vi "Add.vi"(8 "error in (no error)":errorcluster, 9 "Project":refnum<vi>, 10 "IB_Destination.lvclass":refnum<class "IB_Destination.lvclass">, 11 "IB_Tree_Item_Proj in":refnum<class "IB_Tree_Item_Proj.lvclass">) -> (0 "error out":errorcluster, 1 "updated?":bool, 2 "IB_Source.lvclass":refnum<class "IB_Source.lvclass">, 3 "IB_Tree_Item_Proj out":refnum<class "IB_Tree_Item_Proj.lvclass">)   [LabVIEW 2020, in "IB_Tree_Item_Proj.lvclass"]
uses:
  <vilib>/AppBuilder/IB_Classes/Tree_Item_Proj/IB_Tree_Item_Proj.lvclass
  <vilib>/AppBuilder/IB_Classes/Tree_Item_Proj/IB_Tree_Item_Proj.lvclass/IB_Tree_Item_Proj.ctl
  <vilib>/AppBuilder/IB_Classes/Source/IB_Source.lvclass
  <vilib>/AppBuilder/IB_Classes/Destination/IB_Destination.lvclass
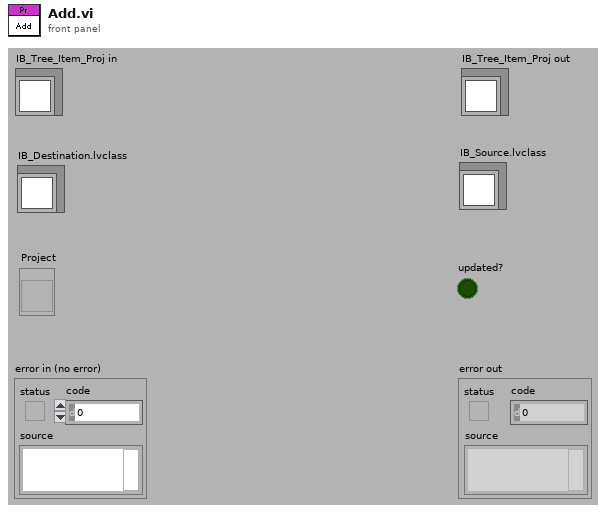
[diagram p1: front panel]
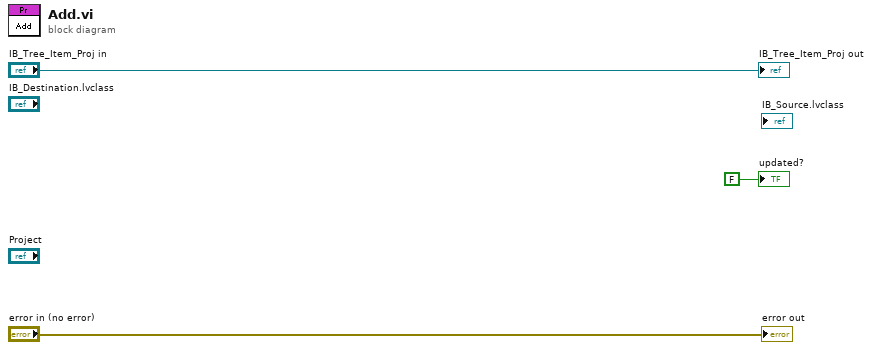
[diagram p0: block diagram]
diagram:
  "error out" <- "error in (no error)"
  "IB_Tree_Item_Proj out" <- "IB_Tree_Item_Proj in"
  "updated?" <- FALSE ("updated?")
